vi "Waveform Buffer Generation (multi).vi"(5 "Amplitude":dbl=2.0 format="%0.2p", 6 "Cycles per Buffer":dbl=1.0 format="%.2f", 7 "Samples per Buffer":dbl=1000.0, 8 "error in":errorcluster caption="error in (no error)", 9 "Waveform Type":u16(ring) items=["Sine Wave", "Triangle Wave", "Square Wave", "Sawtooth Wave"], 10 "Desired Frequency":dbl=1000.0 format="%.2f", 11 "task/channels in":refnum<k21>) -> (0 "error out":errorcluster, 1 "Resulting Frequency":dbl format="%.2f", 2 "Waveform":waveform(dbl)[](array[waveform]), 3 "task out":refnum<k21>, 4 "Resulting Sample Clock Rate":dbl format="%.2f")   [LabVIEW 2022 SP3]
doc: "This subVI is used to create a Sine, Square, Triangle or Sawtooth Waveform. The inputs to this VI are the Waveform Type, which determines if the output waveform is a Sine, Square, Triangle, or Sawtooth Waveform, the amplitude, Desired Frequency, Samples per Buffer, and Cycles per Buffer. \n\nThe Desired Frequency, Samples per Buffer, and Cycles per Buffer are used to calculate the sample clock rate. The DAQmx Timing property node sets the sample clock rate for the device specified in the task/channels in control. \n\nThe actual, coerced, sample clock rate is returned and used as an input to the Basic Function Generator.vi. The Basic Function Generator returns a waveform of data with timing information.\n\nThe formula below was used to determine the sample clock rate:\n\nDesired Frequency=[(Cycles/Buffer)X(Sample Clock Rate)]/Samples per Buffer\n\nNote: The Block Diagram rearranges the variables to solve for Sample Clock Rate"
uses:
  <vilib>/measure/NI_MABase.lvlib
  <resource>/objmgr/daqmx.rc
panel:
  out "Samples/cycle":dbl format="%0.2f"
  out "Desired Sample Clock Rate":dbl format="%.2f"
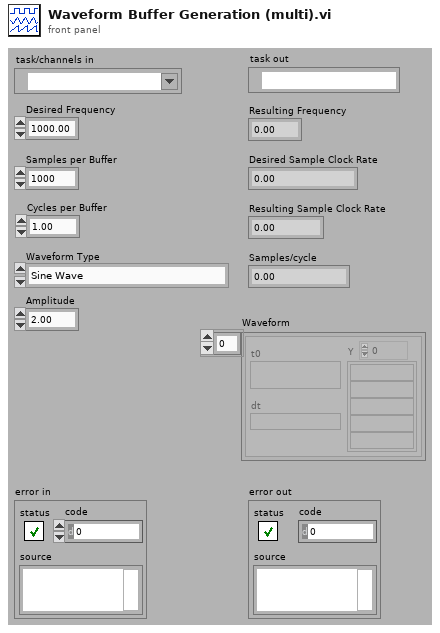
[diagram p1: front panel]
types:
  T1 = cluster{"SampClk.Rate":dbl, "Samples per Buffer":dbl}
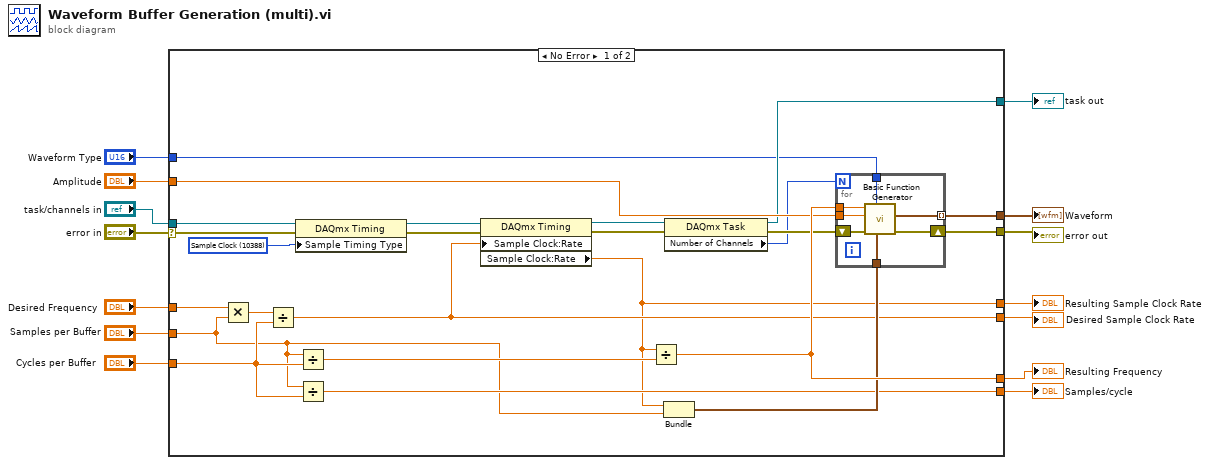
[diagram p0: block diagram]
diagram:
  n1 = case shown="No Error" "error in" {
    selector: "error in" -> [w15 w46]
    tunnel: [w38 _] -> w14
    tunnel: "Desired Frequency" -> [w37 _]
    tunnel: [w34 _] -> w12
    tunnel: "Cycles per Buffer" -> [w33 _]
    tunnel: [w31 _] -> w10
    tunnel: "Amplitude" -> [w30 _]
    tunnel: "Samples per Buffer" -> [w29 _]
    tunnel: [w28 _] -> w7
    tunnel: [w27 w46] -> w6
    tunnel: "task/channels in" -> [w23 w47]
    tunnel: [w19 w47] -> w4
    tunnel: [w18 _] -> w3
    tunnel: "Waveform Type" -> [w17 _]
    frame No Error {
      w24 = 10388 items=["Sample Clock"=10388, "Handshake"=10389, "Implicit"=10451, "On Demand"=10390, "Change Detection"=12504] ("SampTimingType")
      n2 = Multiply(x=w37, y=w29) -> (x*y=w35:dbl)
      n3 = Divide(x=w35, y=w33) -> (x/y=w31:dbl)
      n4 = property class="DAQmx Timing"(reference=w23, error in=w15, "Sample Timing Type"=w24) -> (reference out=w26:refnum<k21>, error out=w25:errorcluster)
      n5 = Divide(x=w29, y=w33) -> (x/y=w32:dbl)
      n6 = Divide(x=w29, y=w33) -> (x/y=w34:dbl)
      n7 = property class="DAQmx Timing"(reference=w26, error in=w25, "Sample Clock:Rate"=w31) -> (reference out=w21:refnum<k21>, error out=w22:errorcluster, "Sample Clock:Rate"=w28:dbl)
      n8 = Divide(x=w28, y=w32) -> (x/y=w38:dbl)
      n9 = Bundle("SampClk.Rate"=w28, "Samples per Buffer"=w29) -> (w36:T1)  [unwired: 1 in]
      n10 = property class="DAQmx Task"(reference=w21, error in=w22) -> (reference out=w19:refnum<k21>, error out=w20:errorcluster, "Number of Channels"=w16:u32)
      n11 = for {
        N: w16 -> [_]
        tunnel: w38 -> [w45]
        tunnel: w36 -> [w44]
        tunnel: [w43] -> w18 mode=indexing
        tunnel: w30 -> [w42]
        shift-right: [w41] -> w27
        shift-left: w20 -> [w40]
        tunnel: w17 -> [w39]
        n12 = call <vilib>:"Basic Function Generator.vi"("sampling info"=w44, "signal type"=w39, "error in (no error)"=w40, "amplitude"=w42, "frequency"=w45) -> ("error out"=w41:errorcluster, "signal out"=w43:waveform(dbl))  [unwired: 4 in, 1 out]
      }
    }
    frame Error {
    }
  }
  "Resulting Sample Clock Rate" <- w7
  "Desired Sample Clock Rate" <- w10
  "Resulting Frequency" <- w14
  "Samples/cycle" <- w12
  "error out" <- w6
  "task out" <- w4
  "Waveform" <- w3
